vi "CreateGraphicsFromImage.vi"(8 "error in (no error)":errorcluster, 11 "LcPictureBox in":refnum<class "LcPictureBox.lvclass">) -> (0 "error out":errorcluster, 1 "Scale":sgl, 2 "Graphics":refnum<k24>, 3 "LcPictureBox out":refnum<class "LcPictureBox.lvclass">, 4 "Offset":cluster{"x":sgl, "y":sgl})   [LabVIEW 2020, in "LcPictureBox.lvclass"]
uses:
  LcPictureBox.lvclass
  System.Drawing
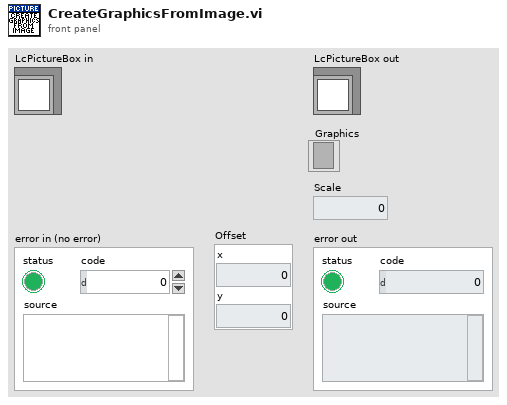
[diagram p1: front panel]
types:
  T1 = typedef "LcPictureBox.lvclass/ObjectAttributes.ctl" = cluster{"PictureBox":refnum<k24>, "ImageSize":cluster{"Width":i32, "Height":i32}, "PenMemory":map{cluster{"Alpha(100%)":dbl, "Color(Black)":u32, "Pen(Width=1, Solid)":T2}, refnum<k24>}, "GraphicsRef":refnum<k24>, "BrushMemory":map{cluster{"Alpha(100%)":dbl, "Color(Black)":u32}, refnum<k24>}, "Images":refnum<k24>[], "ImageIndex":i32, "BgColor(None)":u32, "LoadedImages":map{string, cluster{"ImageOut":refnum<k24>, "ImageSize":cluster{"Width":i32, "Height":i32}}}, "ColorsMemory":map{cluster{"Alpha(100%)":dbl, "Color(Black)":u32}, refnum<k24>}, "CacheSize":i32, "PictureBoxActiveXReference":refnum<vi>, "Scale":sgl, "Offset":cluster{"x":sgl, "y":sgl}, "zoom_center":cluster{"X":i32, "Y":i32}, "ImagesCreated":refnum<k24>[]}
  T2 = typedef "LcPictureBox.lvclass/Pen.ctl" = cluster{"Width":u16, "Style":enum32{"Solid", "Dash", "Dot", "DashDot", "DashDotDot"}}
  T3 = map{cluster{"Alpha(100%)":dbl, "Color(Black)":u32}, refnum<k24>}
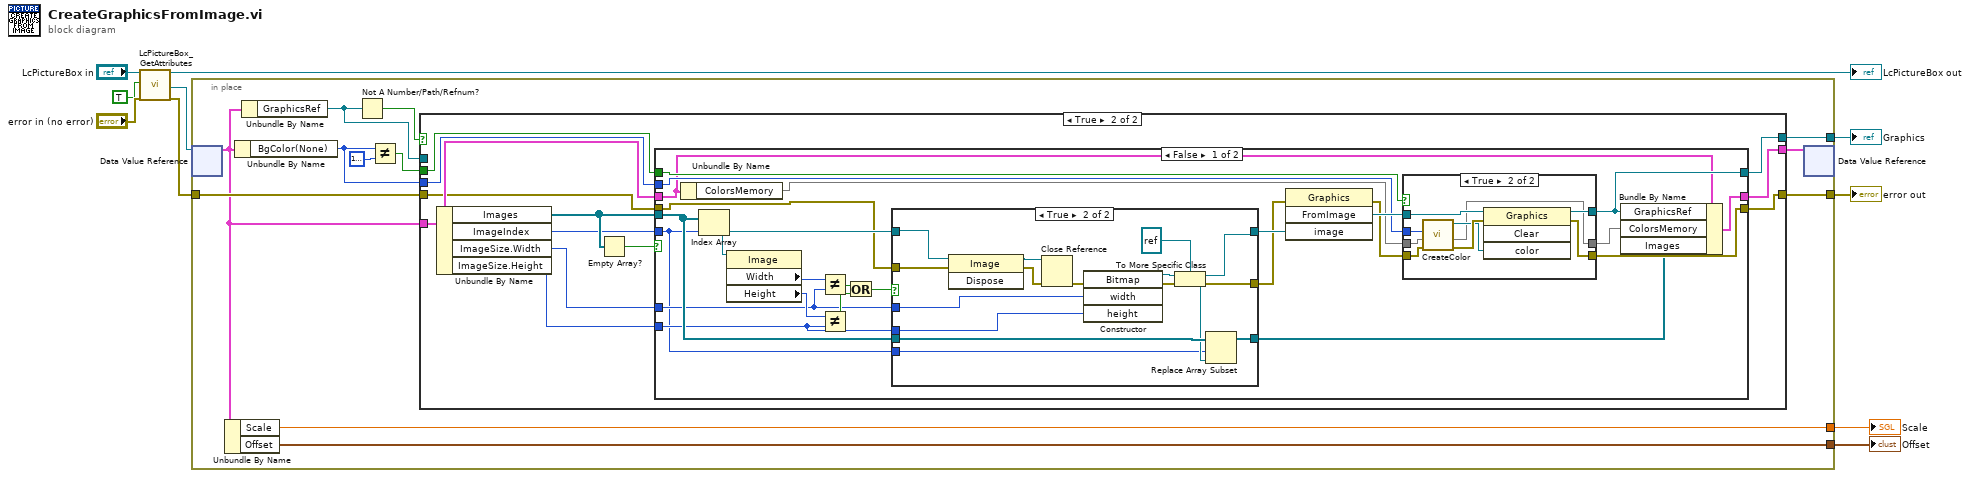
[diagram p0: block diagram]
diagram:
  n1 = call "LcPictureBox_GetAttributes.vi"("reference in"="LcPictureBox in", "OnlyGetDvrReference(False)"=TRUE, "error in (no error)"="error in (no error)") -> ("reference out"=→"LcPictureBox out":refnum<class "LcPictureBox.lvclass">, "DataRef"=w6:refnum<data-value>, "error out"=w5:errorcluster)  [unwired: 13 in, 1 out]
  n2 = in-place {
    in-place-border: w5 -> [w21]
    in-place-border: [w20] -> w4
    in-place-border: [w19] -> w3
    in-place-border: [w12] -> w2
    in-place-border: [w11] -> w1
    n3 = in-place-dvr #1(w6) -> (w13:T1)  [unwired: 1 out]
    n4 = Unbundle By Name(w13) -> ("Scale"=w11:sgl, "Offset"=w12:cluster{"x":sgl, "y":sgl})
    n5 = Unbundle By Name(w13) -> ("BgColor(None)"=w14:u32)
    n6 = Unbundle By Name(w13) -> ("GraphicsRef"=w18:refnum<k24>)
    n7 = Not A Number/Path/Refnum?(number/path/refnum=w18) -> (NaN/Path/Refnum?=w22:bool)
    n8 = Not Equal?(x=w14, y=u32 16777216 ("BgColor(None)")) -> (x != y?=w15:bool)
    n9 = case shown="True" w22 {
      tunnel: w21 -> [w24 w35]
      tunnel: [w24 w34] -> w20
      tunnel: [w25 w33] -> w19
      tunnel: w18 -> [w25 _]
      tunnel: w13 -> [w23 w36]
      tunnel: [w23 w37] -> w17
      tunnel: w15 -> [_ w29]
      tunnel: w14 -> [_ w28]
      frame False {
      }
      frame True {
        n10 = Unbundle By Name(w36) -> ("Images"=w32:refnum<k24>[], "ImageIndex"=w30:i32, "ImageSize.Width"=w27:i32, "ImageSize.Height"=w26:i32)
        n11 = Empty Array?(array=w32) -> (empty?=w31:bool)
        n12 = case shown="False" w31 {
          tunnel: [w61 w92] -> w37
          tunnel: w36 -> [w54 w92]
          tunnel: w35 -> [w41 w93]
          tunnel: [w56 w93] -> w34
          tunnel: [w60 _] -> w33
          tunnel: w32 -> [w44 _]
          tunnel: w30 -> [w38 _]
          tunnel: w29 -> [w58 _]
          tunnel: w28 -> [w55 _]
          tunnel: w27 -> [w40 _]
          tunnel: w26 -> [w39 _]
          frame False {
            n13 = Unbundle By Name(w54) -> ("ColorsMemory"=w53:T3)
            n14 = Index Array(array=w44, index=w38) -> (element=w46:refnum<k24>)
            n15 = property class="Image"(reference=w46) -> ("Width"=w51:i32, "Height"=w50:i32)  [unwired: 1 in, 2 out]
            n16 = Not Equal?(x=w51, y=w40) -> (x != y?=w49:bool)
            n17 = Not Equal?(x=w50, y=w39) -> (x != y?=w48:bool)
            n18 = Or(x=w49, y=w48) -> (x .or. y?=w47:bool)
            n19 = case shown="True" w47 {
              tunnel: w46 -> [w64 w73]
              tunnel: [w64 w66] -> w45
              tunnel: w44 -> [w63 w68]
              tunnel: [w63 w67] -> w43
              tunnel: w41 -> [w62 w72]
              tunnel: [w62 w71] -> w42
              tunnel: w40 -> [_ w70]
              tunnel: w39 -> [_ w69]
              tunnel: w38 -> [_ w65]
              frame False {
              }
              frame True {
                n20 = invoke class="Image" method="Dispose"(reference=w73, error in=w72) -> (reference out=w75:refnum<k24>, error out=w76:errorcluster)  [unwired: 1 in, 1 out]
                n21 = Close Reference(reference=w75, error in (no error)=w76) -> (error out=w77:errorcluster)
                n22 = constructor class="Bitmap"(error in=w77, "width"=w70, "height"=w69) -> (reference out=w79:refnum<k24>, error out=w78:errorcluster)  [unwired: 2 in, 3 out]
                n23 = To More Specific Class(target class=refnum<k24> refnum, reference=w79, error in=w78) -> (specific class reference=w66:refnum<k24>, error out=w71:errorcluster)
                n24 = Replace Array Subset(array=w68, new element=w66, index=w65) -> (w67:refnum<k24>[])
              }
            }
            n25 = invoke class="Graphics" method="FromImage"(error in=w42, "image"=w45) -> (error out=w57:errorcluster, "FromImage"=w59:refnum<k24>)  [unwired: 2 in, 2 out]
            n26 = case shown="True" w58 {
              tunnel: [w81 w91] -> w60
              tunnel: w59 -> [w81 w90]
              tunnel: w57 -> [w82 w89]
              tunnel: [w82 w86] -> w56
              tunnel: w55 -> [_ w87]
              tunnel: w53 -> [w80 w84]
              tunnel: [w80 w83] -> w52
              frame False {
              }
              frame True {
                n27 = call "CreateColor.vi"("error in (no error)"=w89, "ColorsIn"=w84, "Color(Black)"=w87) -> ("error out"=w88:errorcluster, "ColorsOut"=w83:T3, "ColorRef"=w85:refnum<k24>)  [unwired: 6 in]
                n28 = invoke class="Graphics" method="Clear"(reference=w90, error in=w88, "color"=w85) -> (reference out=w91:refnum<k24>, error out=w86:errorcluster)  [unwired: 1 in, 2 out]
              }
            }
            n29 = Bundle By Name(cluster=w54, "GraphicsRef"=w60, "ColorsMemory"=w52, "Images"=w43) -> (w61:T1)
          }
          frame True {
          }
        }
      }
    }
    n30 = in-place-dvr #1(w17) -> ()  [unwired: 2 out]
  }
  "error out" <- w4
  "Graphics" <- w3
  "Scale" <- w1
  "Offset" <- w2
